vi "Add Noise.vi"(6 "Sampling":T1 {"Fs" format="%#_13g"}, 8 "error in (no error)":errorcluster, 11 "AI []":waveform(dbl)[](array[waveform])) -> (0 "error out":errorcluster, 3 "AI + Noise":waveform(dbl)[](array[waveform]))   [LabVIEW 2019, in "DAQmx.lvclass"]
uses:
  DAQmx.lvclass
  Instrument.DAQ/Typedefs/DAQ.Sampling.Sampling--Cluster.ctl
  <vilib>/measure/NI_MAPro.lvlib
  <vilib>/measure/maspectr.llb/FFT Power Spectrum and PSD for N Chan.vi
  Instrument.DAQ/Instrument.DAQ.lvclass
panel:
  out "Waveform Graph":cluster{"f0":dbl, "df":dbl, "magnitude":dbl[]}[](graph)
  in  "Noise Cluster":T2={"1/f vs. Uniform "=1.0, "60Hz Amplitude"=0.005, "Gauss/Unif %"=0.5, "Noise Amp"=0.005}
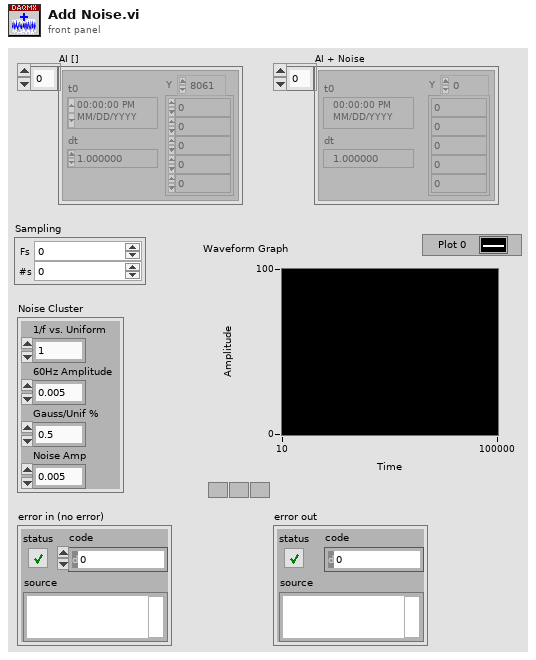
[diagram p1: front panel]
types:
  T1 = typedef "Instrument.Lockin.lvlib/Instrument.DAQ.lvclass/DAQ.Sampling.Sampling--Cluster.ctl" = cluster{"Fs":dbl, "#s":i32}
  T2 = cluster{"1/f vs. Uniform ":dbl, "60Hz Amplitude":dbl, "Gauss/Unif %":dbl, "Noise Amp":dbl}
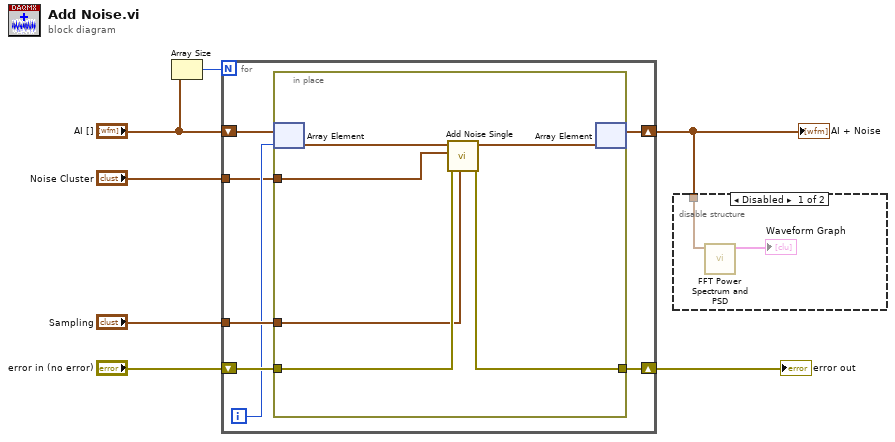
[diagram p0: block diagram]
diagram:
  n1 = Array Size(array="AI []") -> (size(s)=w3:i32)
  n2 = for {
    N: w3 -> [_]
    tunnel: "Noise Cluster" -> [w8]
    tunnel: "Sampling" -> [w14]
    shift-right: [w12] -> w1
    shift-left: "error in (no error)" -> [w13]
    shift-right: [w9] -> w4
    shift-left: "AI []" -> [w11]
    i -> [w10]
    n3 = in-place {
      in-place-border: w14 -> [w16]
      in-place-border: w13 -> [w18]
      in-place-border: [w17] -> w12
      in-place-border: w8 -> [w15]
      n4 = in-place-array #1(w11, w10) -> (w20:waveform(dbl))
      n5 = call "Add Noise Single.vi"("Sampling"=w16, "error in (no error)"=w18, "Noise Cluster"=w15, "signal in"=w20) -> ("error out"=w17:errorcluster, "signal out"=w19:waveform(dbl))  [unwired: 6 in]
      n6 = in-place-array #1(w19) -> (w9:waveform(dbl)[])  [unwired: 1 out]
    }
  }
  "AI + Noise" <- w4
  "error out" <- w1
  n7 = disable-structure shown="Disabled" {
    disable-tunnel: w4 -> [w21 _]
    frame Disabled {
      n8 = call-poly <vilib>:"FFT Power Spectrum and PSD.vi"("time signals"=w21) -> ("Power Spectrum / PSD"=→"Waveform Graph":cluster{"f0":dbl, "df":dbl, "magnitude":dbl[]}[])  [unwired: 7 in, 3 out]
    }
    frame Enabled {
    }
  }
